vi "ConfigureInternalClockSynced.vi"(0 "object in":refnum<class "Hamamatsu.lvclass">, 2 "FramesPerAquisionCycle":i32, 3 "CameraBufferSize":i32, 5 "error in (no error)":errorcluster, 8 "Master pulse Parameters":T1={"Mode"=1, "Source"=1, "Interval"=1.0, "Burst"=0} {"Source" items=["External"=1, "Software"=2]; "Mode" items=["Continuous"=1, "Start"=2, "Burst"=3]}) -> (14 "object out":refnum<class "Hamamatsu.lvclass">, 19 "error out":errorcluster)   [LabVIEW 2024, in "Hamamatsu.lvclass"]
uses:
  Hamamatsu.lvclass
  Hamamatsu.lvclass/Hamamatsu.ctl
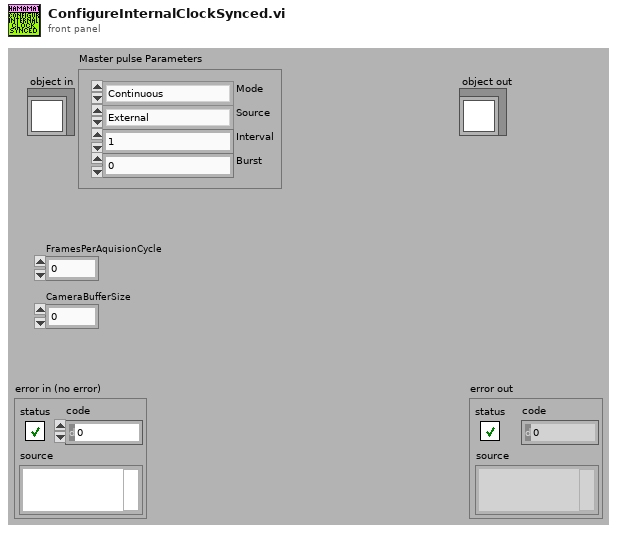
[diagram p1: front panel]
types:
  T1 = cluster{"Mode":u32, "Source":u32, "Interval":dbl, "Burst":u32}
  T2 = typedef "IMAQ Image.ctl" = refnum<image>
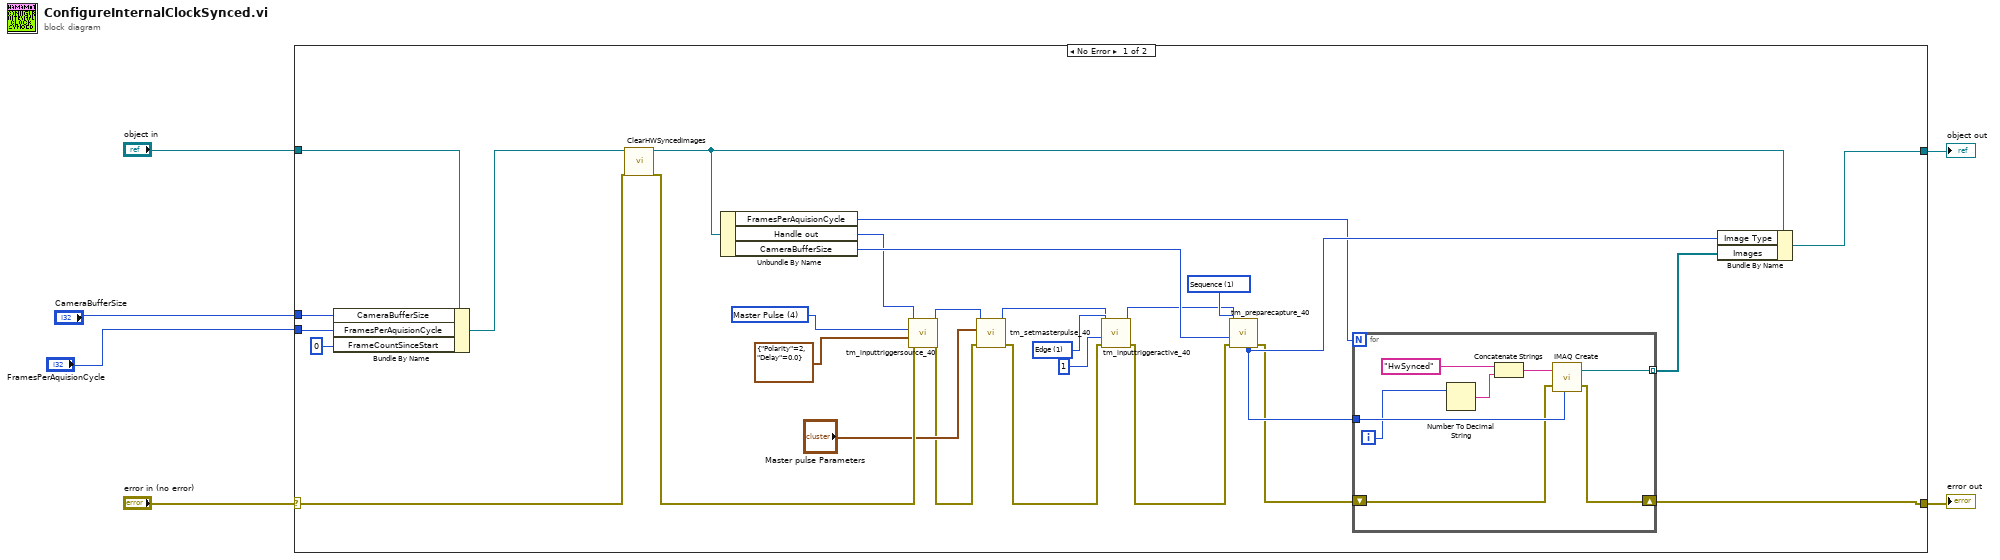
[diagram p0: block diagram]
diagram:
  n1 = case shown="No Error" "error in (no error)" {
    selector: "error in (no error)" -> [w19 w44]
    tunnel: [w29 w44] -> w5
    tunnel: [w30 w43] -> w3
    tunnel: "object in" -> [w14 w43]
    tunnel: "CameraBufferSize" -> [w13 _]
    tunnel: "FramesPerAquisionCycle" -> [w16 _]
    frame No Error {
      w24 = 1 items=["Edge"=1, "Level"=2, "Sync Readout"=3, "Point"=4] ("Active")
      w28 = 4 items=["Internal"=1, "External"=2, "Software"=3, "Master Pulse"=4] ("Source")
      w34 = 1 items=["Snap", "Sequence"] ("Capture mode")
      n2 = Bundle By Name(cluster=w14, "CameraBufferSize"=w13, "FramesPerAquisionCycle"=w16, "FrameCountSinceStart"=0) -> (w15:refnum<class "Hamamatsu.lvclass">)
      n3 = call-dynamic "ClearHWSyncedImages.vi"("object in"=w15, "error in (no error)"=w19) -> ("object out"=w20:refnum<class "Hamamatsu.lvclass">, "error out"=w18:errorcluster)  [unwired: 16 in]
      n4 = Unbundle By Name(w20) -> ("FramesPerAquisionCycle"=w17:i32, "Handle out"=w27:u32, "CameraBufferSize"=w31:i32)
      n5 = call <userlib>:"tm_inputtriggersource_40.vi"("error in (no error)"=w18, "External Options"=cluster{"Polarity":i32, "Delay":dbl} {"Polarity"=2, "Delay"=0.0}, "Source"=w28, "Handle in"=w27) -> ("error out"=w8:errorcluster, "Handle out"=w10:u32)  [unwired: 6 in]
      n6 = call <userlib>:"tm_setmasterpulse_40.vi"("error in (no error)"=w8, "Parameters"="Master pulse Parameters", "Handle in"=w10) -> ("error out"=w7:errorcluster, "Handle out"=w9:u32)  [unwired: 7 in]
      n7 = call <userlib>:"tm_inputtriggeractive_40.vi"("error in (no error)"=w7, "Times"=1, "Active"=w24, "Handle in"=w9) -> ("error out"=w22:errorcluster, "Handle out"=w25:u32)  [unwired: 6 in]
      n8 = call <userlib>:"tm_preparecapture_40.vi"("error in (no error)"=w22, "Frames"=w31, "Capture mode"=w34, "Handle in"=w25) -> ("error out"=w32:errorcluster, "Image type"=w33:u32)  [unwired: 4 in, 2 out]
      n9 = for {
        N: w17 -> [_]
        tunnel: w33 -> [w41]
        shift-right: [w39] -> w29
        shift-left: w32 -> [w40]
        tunnel: [w38] -> w21 mode=indexing
        i -> [w37]
        n10 = Number To Decimal String(number=w37) -> (decimal integer string=w35:string)  [unwired: 1 in]
        n11 = Concatenate Strings("HwSynced" ("Image Name"), w35) -> (w36:string)
        n12 = call "IMAQ Create"("Image Name"=w36, "Image Type"=w41, "error in (no error)"=w40) -> ("New Image"=w38:T2, "error out"=w39:errorcluster)  [unwired: 2 in]
      }
      n13 = Bundle By Name(cluster=w20, "Image Type"=w33, "Images"=w21) -> (w30:refnum<class "Hamamatsu.lvclass">)
    }
    frame Error {
    }
  }
  "error out" <- w5
  "object out" <- w3
